vi "3.vi"() -> ()   [LabVIEW 2020]
panel:
  in  "Length":i32
  out "XY Graph":cluster{i32[], i32[]}(graph)
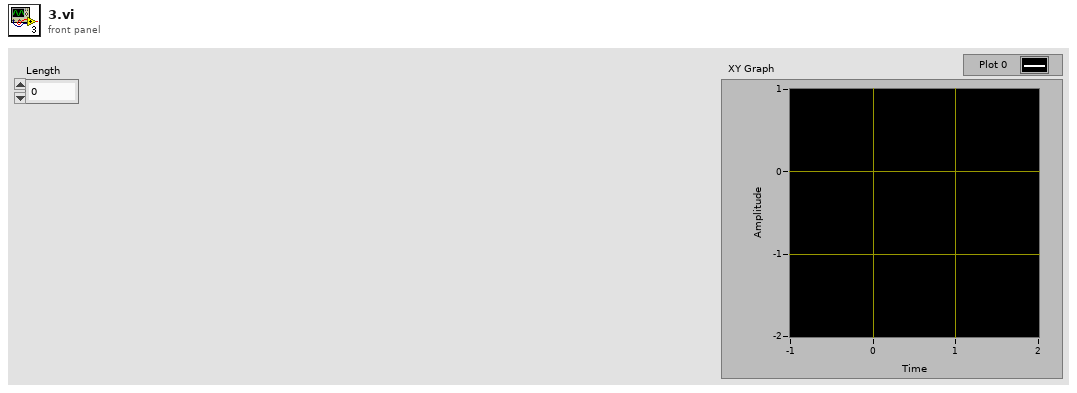
[diagram p1: front panel]
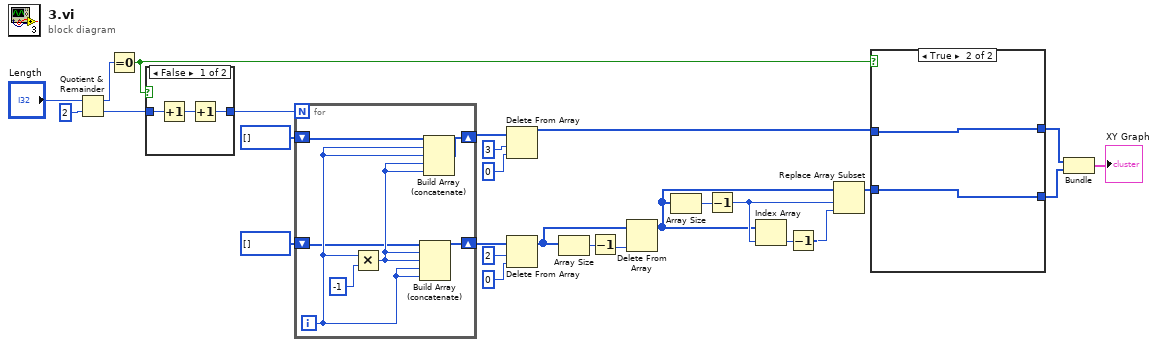
[diagram p0: block diagram]
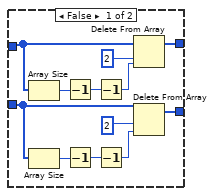
[diagram p2: hidden frame]
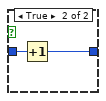
[diagram p3: hidden frame]
diagram:
  n1 = Quotient & Remainder(x="Length", y=2) -> (x-y*floor(x/y)=w6:i32, floor(x/y)=w8:i32)
  n2 = Equal To 0?(x=w6) -> (x = 0?=w5:bool)
  n3 = case shown="False" w5 {
    tunnel: [w28 w32] -> w10
    tunnel: w8 -> [w30 w31]
    frame False {
      n4 = Increment(x=w30) -> (x+1=w29:i32)
      n5 = Increment(x=w29) -> (x+1=w28:i32)
    }
    frame True {
      n6 = Increment(x=w31) -> (x+1=w32:i32)
    }
  }
  n7 = for {
    N: w10 -> [_]
    shift-right: [w38] -> w24
    shift-left: i32[] [] -> [w37]
    shift-right: [w34] -> w19
    shift-left: i32[] [] -> [w33]
    i -> [w35]
    n8 = Multiply(x=w35, y=-1) -> (x*y=w36:i32)
    n9 = Build Array (concatenate)(w33, w36, w36, w35, w35) -> (w34:i32[])
    n10 = Build Array (concatenate)(w37, w35, w35, w36, w36) -> (w38:i32[])
  }
  n11 = Delete From Array(array=w24, length=3, index=0) -> (array with subset deleted=w4:i32[])  [unwired: 1 out]
  n12 = Delete From Array(array=w19, length=2, index=0) -> (array with subset deleted=w17:i32[])  [unwired: 1 out]
  n13 = Array Size(array=w17) -> (size(s)=w18:i32)
  n14 = Decrement(x=w18) -> (x-1=w16:i32)
  n15 = Delete From Array(array=w17, index=w16) -> (array with subset deleted=w11:i32[])  [unwired: 1 in, 1 out]
  n16 = Array Size(array=w11) -> (size(s)=w15:i32)
  n17 = Decrement(x=w15) -> (x-1=w14:i32)
  n18 = Index Array(array=w11, index=w14) -> (element=w13:i32)
  n19 = Decrement(x=w13) -> (x-1=w12:i32)
  n20 = Replace Array Subset(array=w11, new element=w12, index=w14) -> (w1:i32[])
  n21 = case shown="True" w5 {
    tunnel: w4 -> [w42 w53]
    tunnel: [w41 w53] -> w3
    tunnel: [w40 w52] -> w2
    tunnel: w1 -> [w43 w52]
    frame False {
      n22 = Array Size(array=w42) -> (size(s)=w51:i32)
      n23 = Array Size(array=w43) -> (size(s)=w50:i32)
      n24 = Decrement(x=w51) -> (x-1=w45:i32)
      n25 = Decrement(x=w50) -> (x-1=w47:i32)
      n26 = Decrement(x=w45) -> (x-1=w44:i32)
      n27 = Decrement(x=w47) -> (x-1=w46:i32)
      n28 = Delete From Array(array=w42, length=2, index=w44) -> (array with subset deleted=w41:i32[])  [unwired: 1 out]
      n29 = Delete From Array(array=w43, length=2, index=w46) -> (array with subset deleted=w40:i32[])  [unwired: 1 out]
    }
    frame True {
    }
  }
  n30 = Bundle(w3, w2) -> (→"XY Graph":cluster{i32[], i32[]})  [unwired: 1 in]
